vi "Check Out Ref.vi"(8 "error in":errorcluster, 11 "VI Ref":refnum<vi>) -> (0 "error out":errorcluster, 1 "VI Name":string, 2 "Found?":bool, 3 "VI Ref out":refnum<vi>)   [LabVIEW 2015, in "VI.lvlib"]
uses:
  VI.lvlib
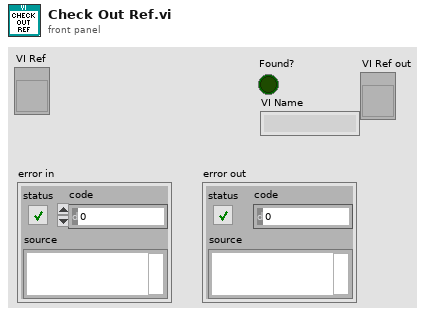
[diagram p1: front panel]
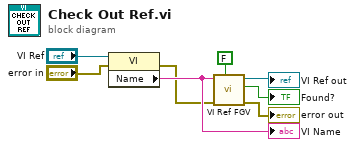
[diagram p0: block diagram]
diagram:
  n1 = property class="VI"(reference="VI Ref", error in="error in") -> (error out=w1:errorcluster, "Name"=w3:string)  [unwired: 1 out]
  "VI Name" <- w3
  n2 = call "VI Ref FGV.vi"("Check in"=FALSE, "error in (no error)"=w1, "Name"=w3) -> ("error out"=→"error out":errorcluster, "Found?"=→"Found?":bool, "Ref out"=→"VI Ref out":refnum<vi>)  [unwired: 6 in]
